vi "status machine.vi"() -> ()   [LabVIEW 2014]
uses:
  status.ctl
panel:
  in  "정지 버튼":bool
  in  "작업 3":bool
  in  "작업 2":bool
  in  "작업 1":bool
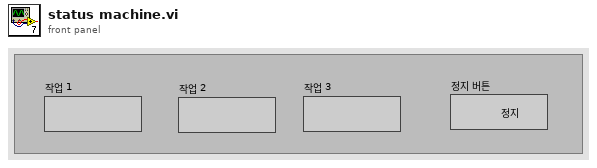
[diagram p1: front panel]
types:
  T1 = typedef "status.ctl" = enum16{"idle", "초기화", "정지", "작업1", "작업2", "작업3"}
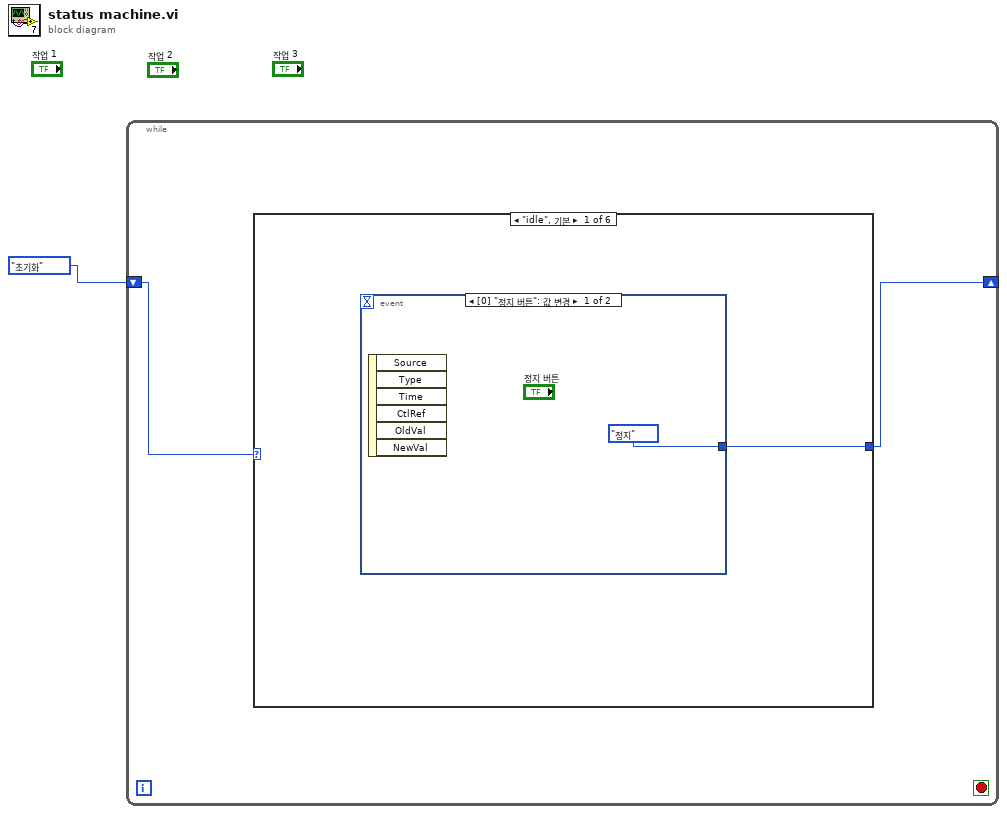
[diagram p0: block diagram]
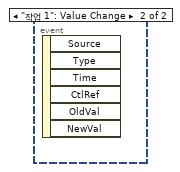
[diagram p2: hidden frame]
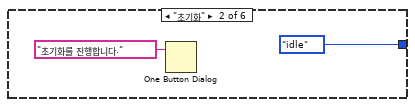
[diagram p3: hidden frame]
diagram:
  n1 = while {
    shift-right: [w2] -> _
    shift-left: status."초기화" ("열거형") -> [w3]
    stop <- _ stop-if-true
    n2 = case shown="\"idle\", 기본" w3 {
      tunnel: [w4 status."idle" ("열거형") _ _ _ _] -> w2
      frame "idle", Default {
        n3 = event shown="[0] \"정지 버튼\": 값 변경" {
          selector: _ -> [_ _]
          dyn-events: _ -> [_ _]
          timeout: _ -> [_ _]
          tunnel: [status."정지" ("열거형") _] -> w4
          event "정지 버튼": Value Change {
            n4 = event-data() -> ()  [unwired: 1 in, 6 out]
          }
          event "작업 1": Value Change {
            n5 = event-data() -> ()  [unwired: 1 in, 6 out]
          }
        }
      }
      frame "초기화" {
        n6 = One Button Dialog(message="초기화를 진행합니다." ("메시지")) -> ()  [unwired: 1 in, 1 out]
      }
      frame "정지" {
      }
      frame "작업1" {
      }
      frame "작업2" {
      }
      frame "작업3" {
      }
    }
  }
